vi "Init.vi"(8 "error in (no error)":errorcluster, 11 "UI Actor in":refnum<class "UI Actor.lvclass">) -> (0 "error out":errorcluster, 3 "UI Actor out":refnum<class "UI Actor.lvclass">)   [LabVIEW 2020, in "UI Actor.lvlib" / "UI Actor.lvclass"]
uses:
  UI Actor.lvclass
  C:/Program Files (x86)/National Instruments/LabVIEW 2020/vi.lib/ActorFramework/Actor/Actor.lvclass
  Messages Actor/Messages Actor.lvclass
  UI Actor.lvclass/UI Actor.ctl
  Nestle Actor/Nestle Actor.lvclass
  Nestle Actor/Nestle Actor.lvclass/Nestle Actor.ctl
  Coca Actor/Coca Actor.lvclass
  Coca Actor/Coca Actor.lvclass/Coca Actor.ctl
  USD Actor/USD Actor.lvclass
  USD Actor/USD Actor.lvclass/USD Actor.ctl
  MXN Actor/MXN Actor.lvclass
  MXN Actor/MXN Actor.lvclass/MXN Actor.ctl
  Messages Actor/Messages Actor.lvclass/Messages Actor.ctl
  Read Coins.vi
  Read Sub Panel monedas.vi
  Read Products.vi
  Read Sub Panel productos.vi
  Read Sub Panel mensajes.vi
  <vilib>/ActorFramework/Actor/Actor.lvclass
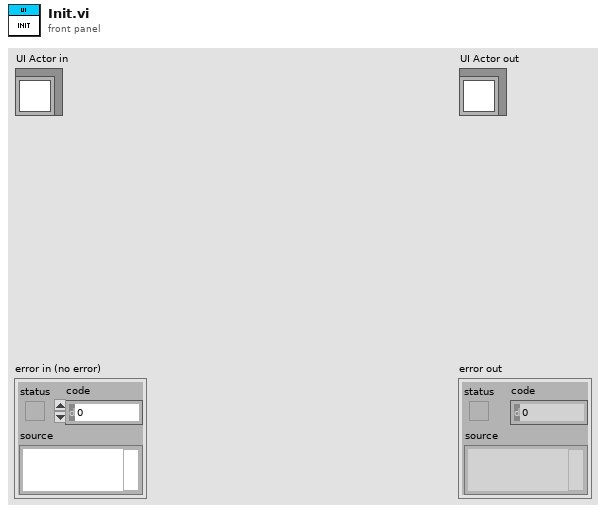
[diagram p1: front panel]
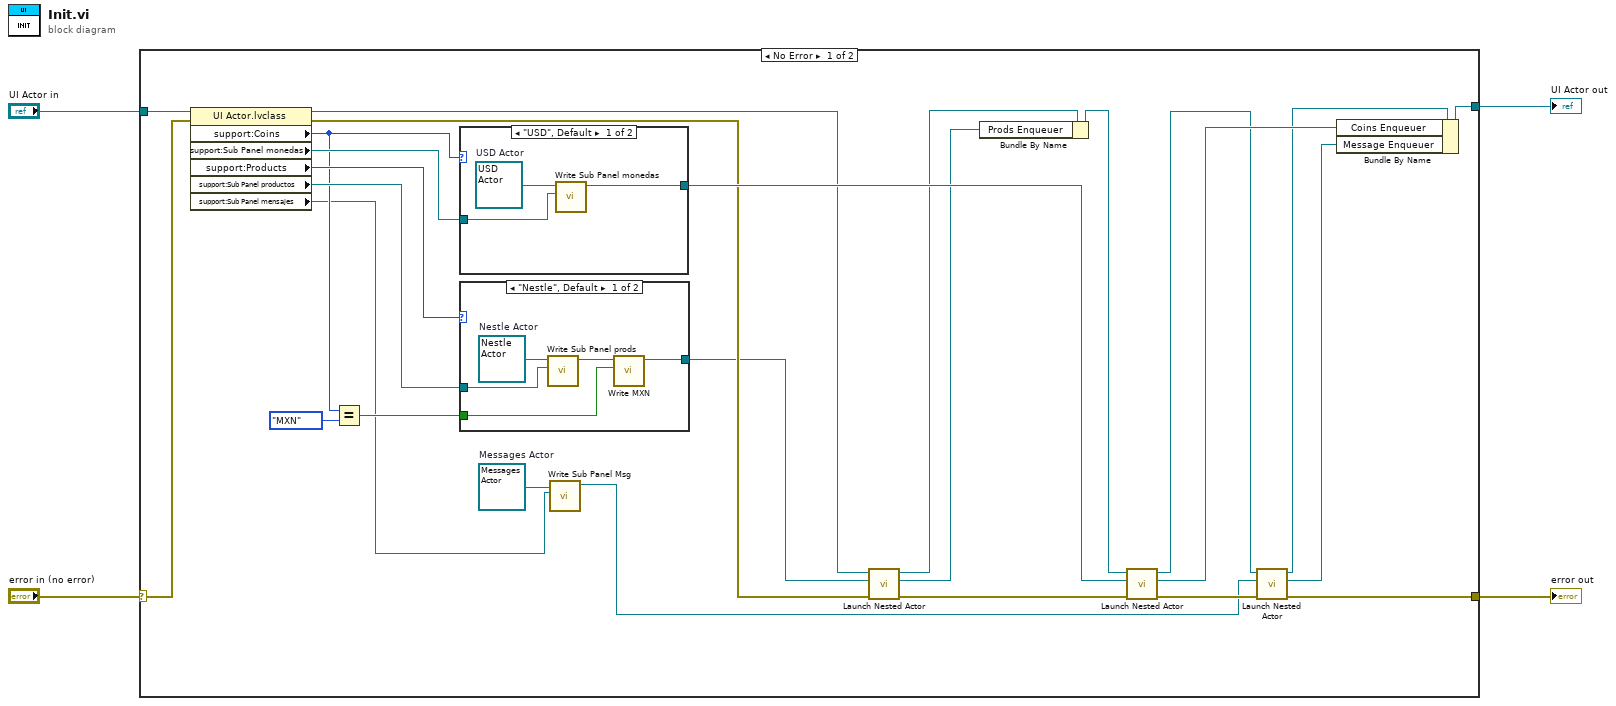
[diagram p0: block diagram]
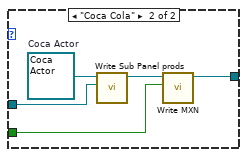
[diagram p2: hidden frame]
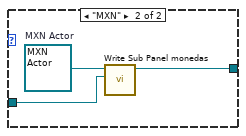
[diagram p3: hidden frame]
diagram:
  n1 = case shown="No Error" "error in (no error)" {
    selector: "error in (no error)" -> [w30 w48]
    tunnel: [w14 w48] -> w3
    tunnel: [w10 w47] -> w1
    tunnel: "UI Actor in" -> [w29 w47]
    frame No Error {
      w16 = refnum<class "Messages Actor.lvclass"> refnum  # Messages Actor
      n2 = property class="UI Actor.lvclass"(reference=w29, error in=w30) -> (reference out=w21:refnum<class "UI Actor.lvclass">, error out=w24:errorcluster, "support:Coins"=w7:enum16{"USD", "MXN"}, "support:Sub Panel monedas"=w26:refnum<vi>, "support:Products"=w25:enum16{"Nestle", "Coca Cola"}, "support:Sub Panel productos"=w19:refnum<vi>, "support:Sub Panel mensajes"=w5:refnum<vi>)
      n3 = Equal?(x=w7, y=enum16{"USD", "MXN"}."MXN") -> (x = y?=w8:bool)
      n4 = case shown="\"USD\", Default" w7 {
        tunnel: [w42 w45] -> w27
        tunnel: w26 -> [w41 w44]
        frame "USD", Default {
          w43 = refnum<class "USD Actor.lvclass"> refnum  # USD Actor
          n5 = call "Write Sub Panel monedas.vi"("Sub Panel monedas"=w41, "USD Actor in"=w43) -> ("USD Actor out"=w42:refnum<class "USD Actor.lvclass">)  [unwired: 8 in, 1 out]
        }
        frame "MXN" {
          w46 = refnum<class "MXN Actor.lvclass"> refnum  # MXN Actor
          n6 = call "Write Sub Panel monedas.vi"("Sub Panel monedas"=w44, "MXN Actor in"=w46) -> ("MXN Actor out"=w45:refnum<class "MXN Actor.lvclass">)  [unwired: 8 in, 1 out]
        }
      }
      n7 = case shown="\"Nestle\", Default" w25 {
        tunnel: [w32 w37] -> w20
        tunnel: w19 -> [w34 w39]
        tunnel: w8 -> [w31 w36]
        frame "Nestle", Default {
          w35 = refnum<class "Nestle Actor.lvclass"> refnum  # Nestle Actor
          n8 = call "Write Sub Panel prods.vi"("Sub Panel prods"=w34, "Nestle Actor in"=w35) -> ("Nestle Actor out"=w33:refnum<class "Nestle Actor.lvclass">)  [unwired: 8 in, 1 out]
          n9 = call "Write MXN.vi"("MXN"=w31, "Nestle Actor in"=w33) -> ("Nestle Actor out"=w32:refnum<class "Nestle Actor.lvclass">)  [unwired: 8 in, 1 out]
        }
        frame "Coca Cola" {
          w40 = refnum<class "Coca Actor.lvclass"> refnum  # Coca Actor
          n10 = call "Write Sub Panel prods.vi"("Sub Panel prods"=w39, "Coca Actor in"=w40) -> ("Coca Actor out"=w38:refnum<class "Coca Actor.lvclass">)  [unwired: 8 in, 1 out]
          n11 = call "Write MXN.vi"("MXN"=w36, "Coca Actor in"=w38) -> ("Coca Actor out"=w37:refnum<class "Coca Actor.lvclass">)  [unwired: 8 in, 1 out]
        }
      }
      n12 = call "Write Sub Panel Msg.vi"("Sub Panel Msg"=w5, "Messages Actor in"=w16) -> ("Messages Actor out"=w13:refnum<class "Messages Actor.lvclass">)  [unwired: 8 in, 1 out]
      n13 = call <vilib>:"Launch Nested Actor.vi"("error in (no error)"=w24, "Nested Actor"=w20, "Caller Actor in"=w21) -> ("error out"=w23:errorcluster, "Nested Actor's Enqueuer"=w17:refnum<class "Message Enqueuer.lvclass">, "Caller Actor out"=w22:refnum<class "UI Actor.lvclass">)  [unwired: 6 in]
      n14 = Bundle By Name(cluster=w22, "Prods Enqueuer"=w17) -> (w18:refnum<class "UI Actor.lvclass">)
      n15 = call <vilib>:"Launch Nested Actor.vi"("error in (no error)"=w23, "Nested Actor"=w27, "Caller Actor in"=w18) -> ("error out"=w15:errorcluster, "Nested Actor's Enqueuer"=w28:refnum<class "Message Enqueuer.lvclass">, "Caller Actor out"=w12:refnum<class "UI Actor.lvclass">)  [unwired: 6 in]
      n16 = call <vilib>:"Launch Nested Actor.vi"("error in (no error)"=w15, "Nested Actor"=w13, "Caller Actor in"=w12) -> ("error out"=w14:errorcluster, "Nested Actor's Enqueuer"=w9:refnum<class "Message Enqueuer.lvclass">, "Caller Actor out"=w11:refnum<class "UI Actor.lvclass">)  [unwired: 6 in]
      n17 = Bundle By Name(cluster=w11, "Coins Enqueuer"=w28, "Message Enqueuer"=w9) -> (w10:refnum<class "UI Actor.lvclass">)
    }
    frame Error {
    }
  }
  "error out" <- w3
  "UI Actor out" <- w1
